vi "init.vi"(8 "error in (no error)":errorcluster, 11 "Logger in":refnum<class "Logger.lvclass">) -> (0 "error out":errorcluster, 3 "Logger out":refnum<class "Logger.lvclass">)   [LabVIEW 2013, in "Logger.lvclass"]
uses:
  Logger.lvclass
  Configuration/System Controller.ctl
  Configuration/PIDGains.ctl
  Logger.lvclass/Logger.ctl
  ConfigurationThisComponent/ConfigurationThisComponent.lvclass
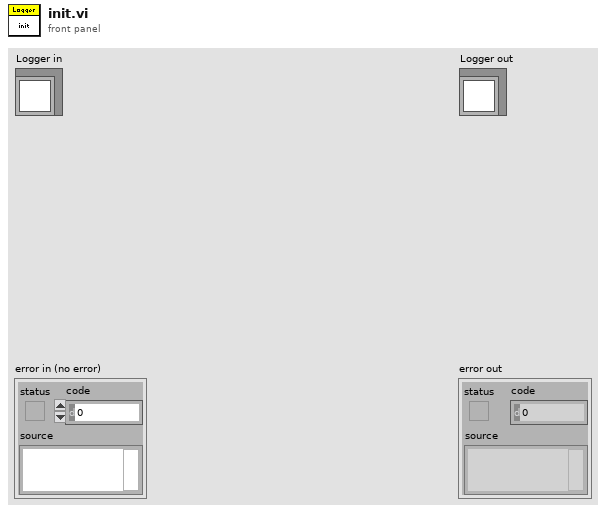
[diagram p1: front panel]
types:
  T1 = typedef "System Controller.ctl" = cluster{"PID Gains":T2, "Force Error In Range Limit":dbl[unit]}
  T2 = typedef "PIDGains.ctl" = cluster{"Proportional Gain (Kc)":dbl, "Integral Time (Ti, min)":dbl, "Derivative Time (Td, min)":dbl}
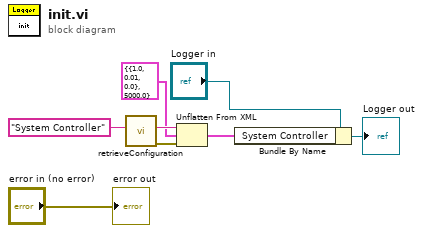
[diagram p0: block diagram]
diagram:
  n1 = call "retrieveConfiguration.vi"("configName"="System Controller") -> ("error out"=w6:errorcluster, "xmlConfig"=w5:string)  [unwired: 8 in, 1 out]
  n2 = Unflatten From XML(xml string=w5, type=T1 {"PID Gains"={"Proportional Gain (Kc)"=1.0, "Integral Time (Ti, min)"=0.01, "Derivative Time (Td, min)"=0.0}, "Force Error In Range Limit"=5000.0} ("System Controller"), error in (no error)=w6) -> (value=w3:T1)  [unwired: 1 out]
  n3 = Bundle By Name(cluster="Logger in", "System Controller"=w3) -> (→"Logger out":refnum<class "Logger.lvclass">)
  "error out" <- "error in (no error)"
